vi "replace_ego_spawn_position.vi"(4 "Start location":dbl[](array[numeric]), 5 "Start rotation":dbl[](array[numeric]), 6 "error in":errorcluster, 8 "Cluster":T2, 9 "vehicles":T1(array[cluster])) -> (0 "error out":errorcluster, 3 "vehicles out":T1(array[cluster]))   [LabVIEW 2019]
doc: "Replace the start position and pose of the ego vehicle using the information from the starting position selected by the user"
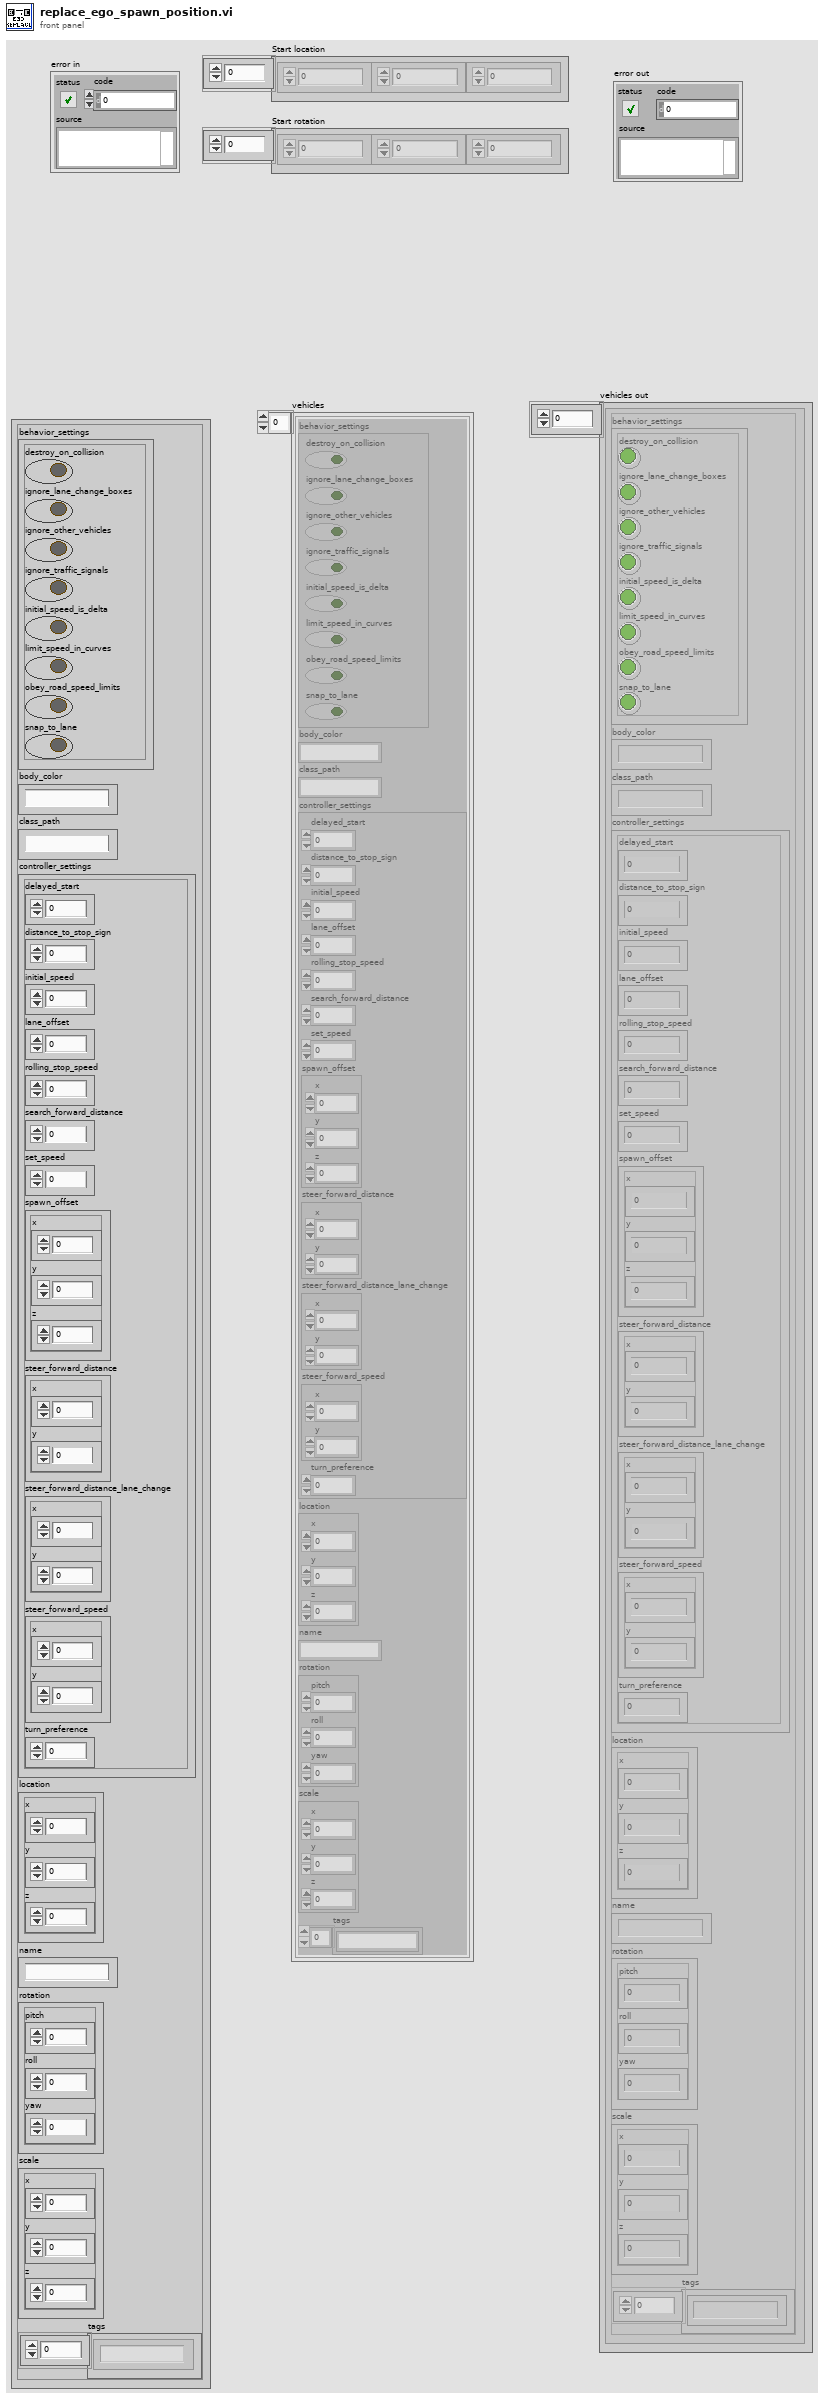
[diagram p1: front panel]
types:
  T1 = cluster{"behavior_settings":cluster{"destroy_on_collision":bool, "ignore_lane_change_boxes":bool, "ignore_other_vehicles":bool, "ignore_traffic_signals":bool, "initial_speed_is_delta":bool, "limit_speed_in_curves":bool, "obey_road_speed_limits":bool, "snap_to_lane":bool}, "body_color":string, "class_path":string, "controller_settings":cluster{"delayed_start":i32, "distance_to_stop_sign":i32, "initial_speed":i32, "lane_offset":i32, "rolling_stop_speed":i32, "search_forward_distance":i32, "set_speed":i32, "spawn_offset":cluster{"x":i32, "y":i32, "z":i32}, "steer_forward_distance":cluster{"x":i32, "y":i32}, "steer_forward_distance_lane_change":cluster{"x":i32, "y":i32}, "steer_forward_speed":cluster{"x":i32, "y":i32}, "turn_preference":i32}, "location":cluster{"x":dbl, "y":i32, "z":i32}, "name":string, "rotation":cluster{"pitch":i32, "roll":i32, "yaw":i32}, "scale":cluster{"x":i32, "y":i32, "z":i32}, "tags":string[]}[]
  T2 = cluster{"behavior_settings":cluster{"destroy_on_collision":bool, "ignore_lane_change_boxes":bool, "ignore_other_vehicles":bool, "ignore_traffic_signals":bool, "initial_speed_is_delta":bool, "limit_speed_in_curves":bool, "obey_road_speed_limits":bool, "snap_to_lane":bool}, "body_color":string, "class_path":string, "controller_settings":cluster{"delayed_start":i32, "distance_to_stop_sign":i32, "initial_speed":i32, "lane_offset":i32, "rolling_stop_speed":i32, "search_forward_distance":i32, "set_speed":i32, "spawn_offset":cluster{"x":i32, "y":i32, "z":i32}, "steer_forward_distance":cluster{"x":i32, "y":i32}, "steer_forward_distance_lane_change":cluster{"x":i32, "y":i32}, "steer_forward_speed":cluster{"x":i32, "y":i32}, "turn_preference":i32}, "location":cluster{"x":dbl, "y":i32, "z":i32}, "name":string, "rotation":cluster{"pitch":i32, "roll":i32, "yaw":i32}, "scale":cluster{"x":i32, "y":i32, "z":i32}, "tags":string[]}
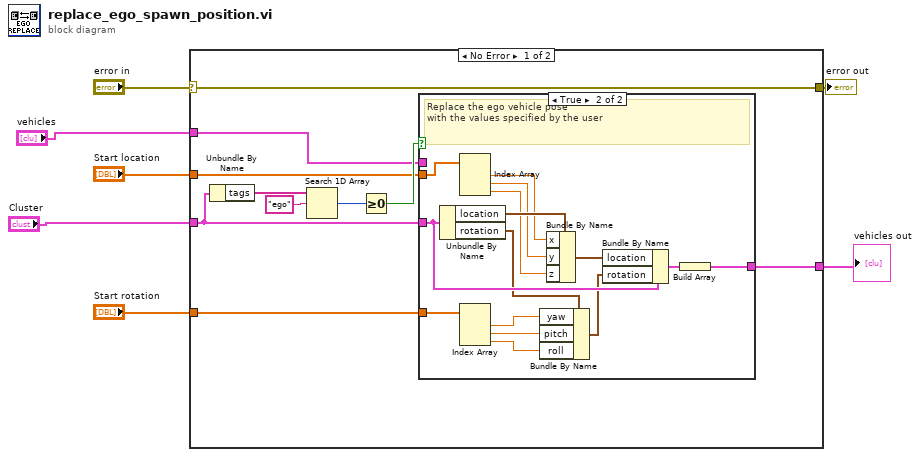
[diagram p0: block diagram]
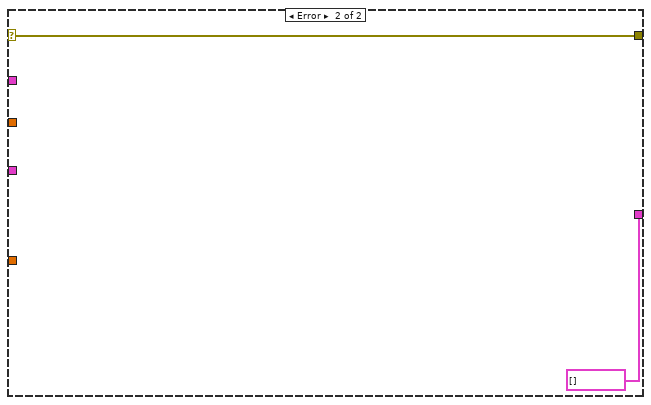
[diagram p3: hidden frame]
diagram:
  n1 = case shown="No Error" "error in" {
    selector: "error in" -> [w12 w35]
    tunnel: "Cluster" -> [w13 _]
    tunnel: [w12 w35] -> w6
    tunnel: "Start location" -> [w11 _]
    tunnel: "Start rotation" -> [w10 _]
    tunnel: "vehicles" -> [w9 _]
    tunnel: [w8 T1 [] ("vehicles")] -> w1
    frame No Error {
      n2 = Unbundle By Name(w13) -> ("tags"=w14:string[])
      n3 = Search 1D Array(1D array=w14, element="ego") -> (index of element=w16:i32)  [unwired: 1 in]
      n4 = Greater Or Equal To 0?(x=w16) -> (x >= 0?=w17:bool)
      n5 = case shown="True" w17 {
        tunnel: w13 -> [_ w33]
        tunnel: w10 -> [_ w30]
        tunnel: w11 -> [_ w24]
        tunnel: [w18 w19] -> w8
        tunnel: w9 -> [w18 _]
        frame False {
          # "Do not change the other verhicles pose"
        }
        frame True {
          # "Replace the ego vehicle pose \nwith the values specified by the user"
          n6 = Unbundle By Name(w33) -> ("location"=w25:cluster{"x":dbl, "y":i32, "z":i32}, "rotation"=w26:cluster{"pitch":i32, "roll":i32, "yaw":i32})
          n7 = Index Array(array=w24) -> (element #1=w23:dbl, element #2=w22:dbl, element #3=w21:dbl)  [unwired: 3 in]
          n8 = Index Array(array=w30) -> (element #1=w29:dbl, element #2=w28:dbl, element #3=w27:dbl)  [unwired: 3 in]
          n9 = Bundle By Name(cluster=w26, "yaw"=w29, "pitch"=w28, "roll"=w27) -> (w31:cluster{"pitch":i32, "roll":i32, "yaw":i32})
          n10 = Bundle By Name(cluster=w25, "x"=w23, "y"=w22, "z"=w21) -> (w20:cluster{"x":dbl, "y":i32, "z":i32})
          n11 = Bundle By Name(cluster=w33, "location"=w20, "rotation"=w31) -> (w32:T2)
          n12 = Build Array(w32) -> (w19:T1)
        }
      }
    }
    frame Error {
    }
  }
  "error out" <- w6
  "vehicles out" <- w1
